vi "DAQNavi Read (Counter 2D Frequency NChan NSamp).vi"(8 "error in (no error)":errorcluster, 9 "number of samples per channel to read":u32=10, 10 "timeout":dbl=10.0, 11 "task in":i32) -> (0 "error out":errorcluster, 2 "data":dbl[][](array[numeric]), 3 "task out":i32)   [LabVIEW 2020]
uses:
  DAQNavi_LV.dll
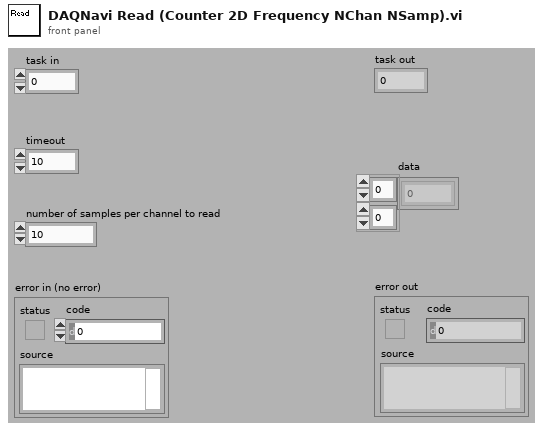
[diagram p1: front panel]
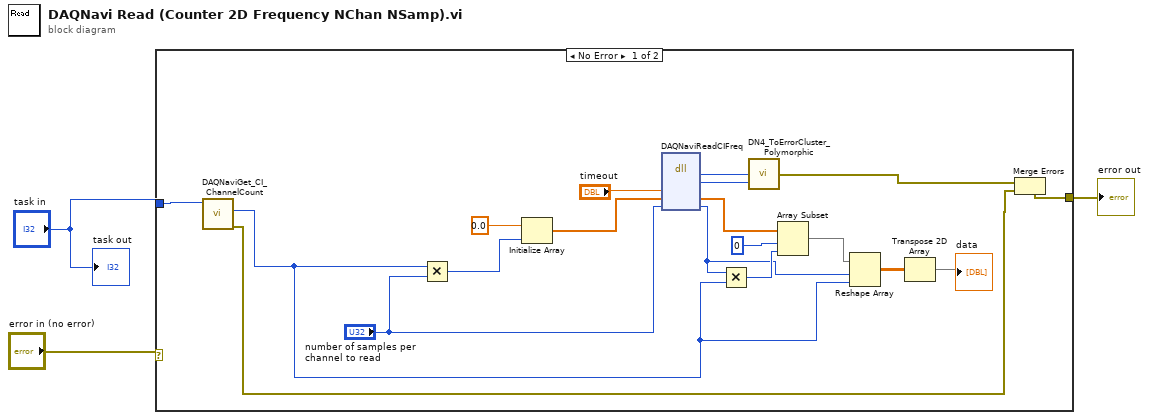
[diagram p0: block diagram]
diagram:
  n1 = case shown="No Error" "error in (no error)" {
    selector: "error in (no error)" -> [_ w23]
    tunnel: "task in" -> [w16 _]
    tunnel: [w7 w23] -> w1
    frame No Error {
      n2 = call "DAQNaviGet_CI_ChannelCount.vi"("task in"=w16) -> ("error out"=w4:errorcluster, "channel count"=w10:i32)  [unwired: 1 in, 8 out]
      n3 = Multiply(x=w10, y="number of samples per channel to read") -> (x*y=w14:u32)
      n4 = Initialize Array(0.0 ("element"), w14) -> (w18:dbl[])
      n5 = dll-call lib="DAQNavi_LV.dll" fn="DAQNaviReadCIFreq"("timeout"="timeout", "freq"=w18, "samples"="number of samples per channel to read") -> ("return type"=w5:i32, "taskID"=w17:i32, "freq"=w21:dbl[], "samples"=w11:u32)  [unwired: 4 in, 3 out]
      n6 = Multiply(x=w11, y=w10) -> (x*y=w13:u32)
      n7 = call "DN4_ToErrorCluster_Polymorphic.vi"("task id"=w17, "error code"=w5) -> ("error out"=w6:errorcluster)  [unwired: 3 out]
      n8 = Array Subset(array=w21, index=0, length=w13) -> (w12:dbl[])
      n9 = Reshape Array(w12, w11, w10) -> (w9:dbl[][])
      n10 = Transpose 2D Array(2D array=w9) -> (transposed array=→"data":dbl[][])
      n11 = Merge Errors(w6, w4) -> (w7:errorcluster)
    }
    frame Error {
    }
  }
  "error out" <- w1
  "task out" <- "task in"
